vi "Inspect Banana.vi"(8 "error in":errorcluster, 11 "Variety Configured":string) -> (0 "error out":errorcluster, 2 "Ephemeral Strategies":string[](array[string]), 3 "Variety":string)   [LabVIEW 2021, in "Bananas.lvlib"]
uses:
  Bananas.lvlib
  Banana/Banana.lvclass/Banana.ctl
  Banana/Banana.lvclass
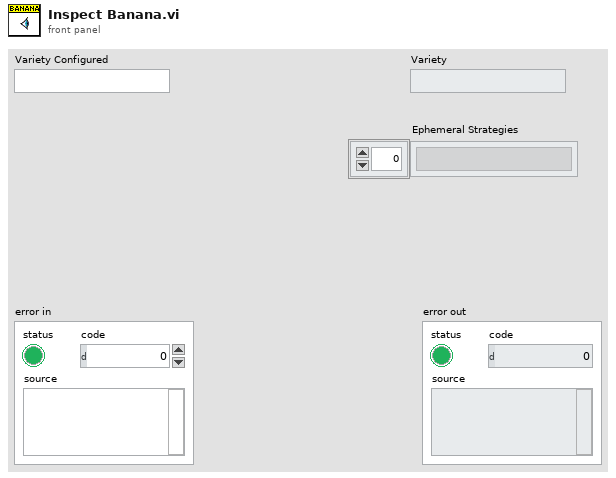
[diagram p1: front panel]
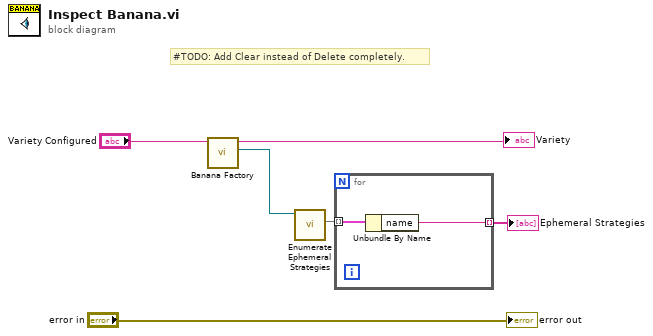
[diagram p0: block diagram]
diagram:
  # "#TODO: Add Clear instead of Delete completely."
  n1 = call "Banana Factory.vi"("Variety"="Variety Configured") -> ("Bunch"=w3:refnum<class "Banana.lvclass">, "Variety Configured"=→"Variety":string)  [unwired: 9 in]
  n2 = call "Enumerate Ephemeral Strategies.vi"("Banana in"=w3) -> ("Ephemerals"=w2:map{string, refnum<class "BananaPeel.lvclass">})  [unwired: 9 in, 1 out]
  n3 = for {
    tunnel: w2 -> [w8] mode=indexing
    tunnel: [w7] -> w1 mode=indexing
    n4 = Unbundle By Name(w8) -> ("name"=w7:string)
  }
  "Ephemeral Strategies" <- w1
  "error out" <- "error in"
